vi "Run.vi"(6 "Type Y":T2(ring), 7 "Type X":T2(ring), 8 "error in (no error)":errorcluster caption="entrée d'erreur (pas d'erreur)", 9 "Y":string[][](array[string]), 10 "X":string[][](array[string]), 11 "Cosine_distances.lvclass":refnum<class "Cosine_distances.lvclass">) -> (0 "error out":errorcluster caption="sortie d'erreur", 2 "Data":T1, 3 "Cosine_distances.lvclass":refnum<class "Cosine_distances.lvclass">)   [LabVIEW 2020, in "Cosine_distances.lvclass"]
doc: "Returns : \n\n- distance matrix : array\nAn array with shape (n_samples_X, n_samples_Y)."
uses:
  Cosine_distances.lvclass
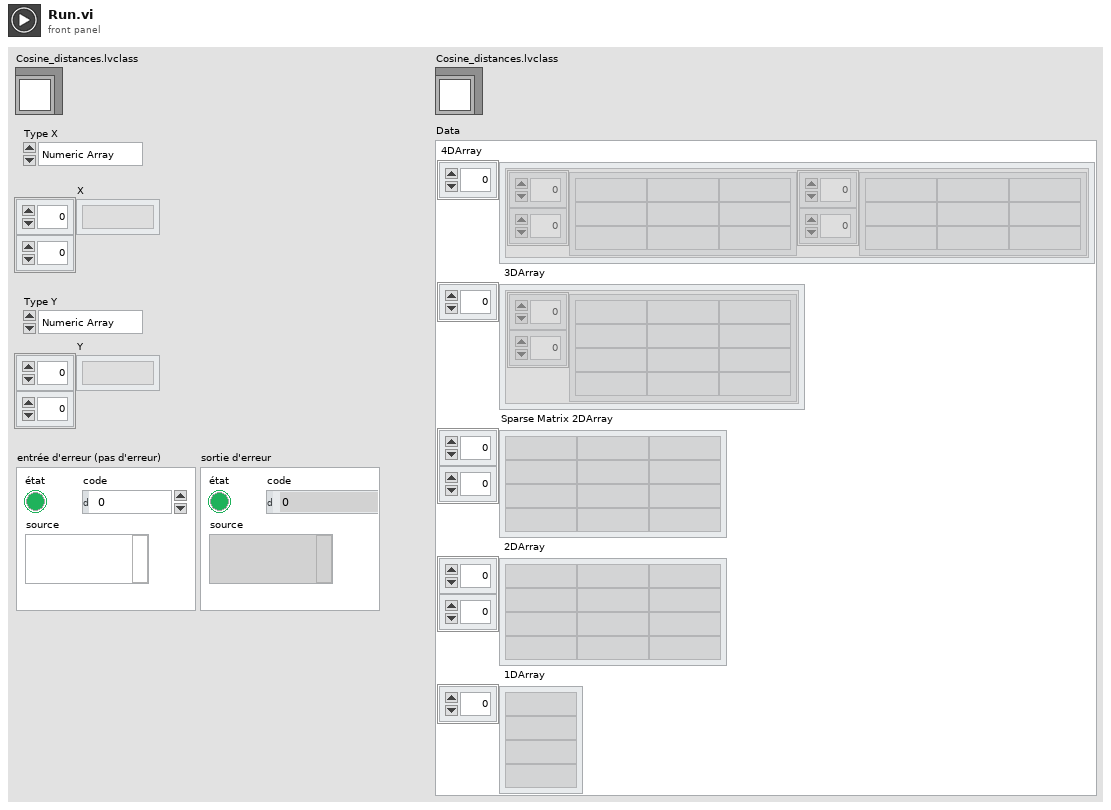
[diagram p1: front panel]
types:
  T1 = cluster{" 4DArray":cluster{"1":string[][], "2":string[][]}[], " 3DArray":cluster{"Tableau":string[][]}[], "Sparse Matrix 2DArray":string[][], " 2DArray":string[][], " 1DArray":string[]}
  T2 = enum16{"Numeric Array", "String Array", "Sparse"}
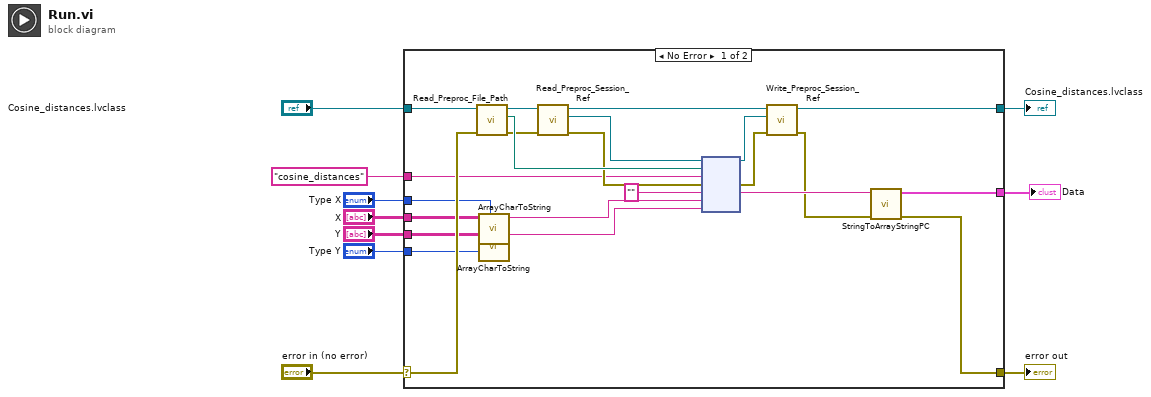
[diagram p0: block diagram]
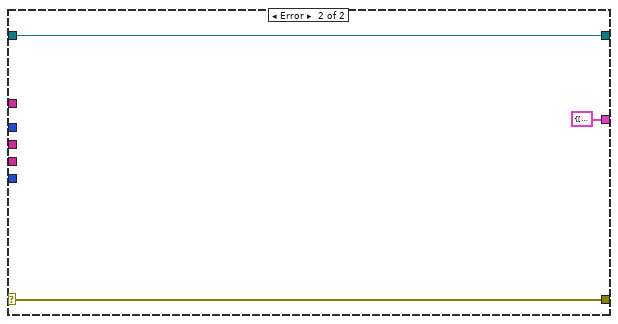
[diagram p2: hidden frame]
diagram:
  n1 = case shown="No Error" "error in (no error)" {
    selector: "error in (no error)" -> [w24 w36]
    tunnel: [w11 w36] -> w9
    tunnel: [w14 w35] -> w7
    tunnel: "Cosine_distances.lvclass" -> [w22 w35]
    tunnel: "cosine_distances" ("Fonction") -> [w23 _]
    tunnel: "X" -> [w21 _]
    tunnel: "Type X" -> [w19 _]
    tunnel: "Y" -> [w18 _]
    tunnel: "Type Y" -> [w16 _]
    tunnel: [w12 T1 {" 4DArray"=[], " 3DArray"=[], "Sparse Matrix 2DArray"=[], " 2DArray"=[], " 1DArray"=[]} ("Data")] -> w1
    frame No Error {
      n2 = call-dynamic "Read_Preproc_File_Path.vi"("error in (no error)"=w24, "Python in"=w22) -> ("error out"=w28:errorcluster, "File_Path"=w31:path, "Python out"=w33:refnum<class "Cosine_distances.lvclass">)  [unwired: 7 in]
      n3 = call "ArrayCharToString.vi"("Type"=w19, "TAB"=w21) -> ("Instruction"=w20:string)  [unwired: 9 in]
      n4 = call "ArrayCharToString.vi"("Type"=w16, "TAB"=w18) -> ("Instruction"=w17:string)  [unwired: 9 in]
      n5 = call-dynamic "Read_Preproc_Session_Ref.vi"("error in (no error)"=w28, "Python in"=w33) -> ("error out"=w29:errorcluster, "Session_ref"=w30:refnum<k35>, "Python out"=w32:refnum<class "Cosine_distances.lvclass">)  [unwired: 7 in]
      n6 = node(w30, w31, w23, w29, "", w20, w17) -> (w25:refnum<k35>, w27:errorcluster, w15:string)  [unwired: 2 in, 2 out]
      n7 = call-dynamic "Write_Preproc_Session_Ref.vi"("error in (no error)"=w27, "Session_ref"=w25, "Python in"=w32) -> ("error out"=w13:errorcluster, "Python out"=w14:refnum<class "Cosine_distances.lvclass">)  [unwired: 7 in]
      n8 = call "StringToArrayStringPC.vi"("sortie d'erreur"=w13, "Return value"=w15) -> ("sortie d'erreur"=w11:errorcluster, "Data"=w12:T1)  [unwired: 8 in]
    }
    frame Error {
    }
  }
  "error out" <- w9
  "Cosine_distances.lvclass" <- w7
  "Data" <- w1
